vi "Series_ejes_flota.vi"(5 "Tabla_flota":string[][](array[string]), 6 "Tags":string[](array[string])) -> (0 "Nº Ejes":i32[](array[numeric]), 1 "Series del convoy":string[](array[string]), 4 "UT":i32[](array[numeric]))   [LabVIEW 2015]
panel:
  out "Array 2":i32[](array[numeric])
  out "Array":i32[](array[numeric])
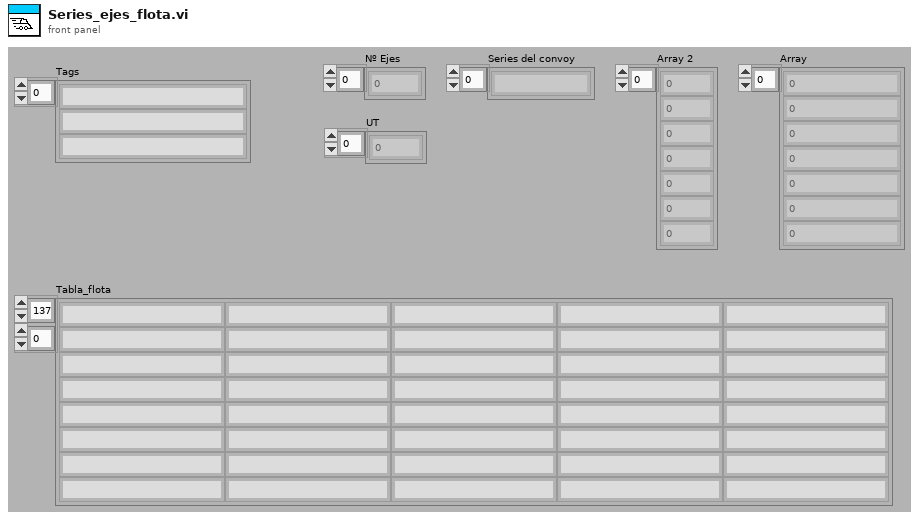
[diagram p1: front panel]
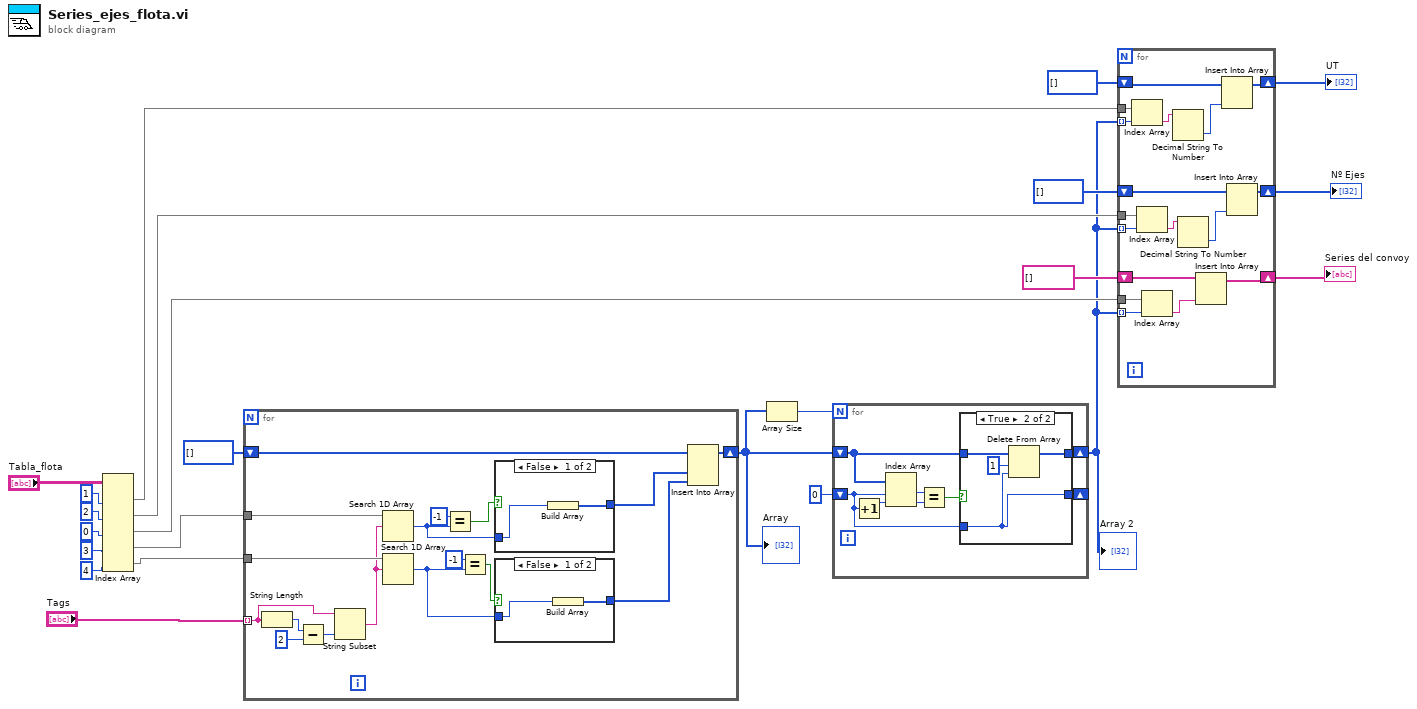
[diagram p0: block diagram]
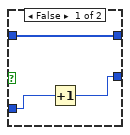
[diagram p2: hidden frame]
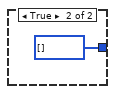
[diagram p3: hidden frame]
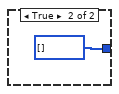
[diagram p4: hidden frame]
diagram:
  n1 = Index Array(array="Tabla_flota", index (col) #1=1 ("index (row)"), index (col) #2=2 ("disabled index (col)"), index (col) #3=0 ("disabled index (col)"), index (col) #4=3 ("disabled index (col)"), index (col) #5=4 ("index (col)")) -> (element #1=w5:string[], element #2=w20:string[], element #3=w17:string[], element #4=w10:string[], element #5=w11:string[])  [unwired: 5 in]
  n2 = for {
    tunnel: "Tags" -> [w28] mode=indexing
    tunnel: w10 -> [w40]
    tunnel: w11 -> [w39]
    shift-right: [w37] -> w13
    shift-left: i32[] [] -> [w38]
    n3 = String Length(string=w28) -> (length=w25:i32)
    n4 = Subtract(x=w25, y=2) -> (x-y=w26:i32)
    n5 = String Subset(string=w28, length (rest)=w26) -> (substring=w27:string)  [unwired: 1 in]
    n6 = Search 1D Array(1D array=w40, element=w27) -> (index of element=w30:i32)  [unwired: 1 in]
    n7 = Search 1D Array(1D array=w39, element=w27) -> (index of element=w29:i32)  [unwired: 1 in]
    n8 = Equal?(x=-1, y=w30) -> (x = y?=w34:bool)
    n9 = Equal?(x=-1, y=w29) -> (x = y?=w33:bool)
    n10 = case shown="False" w34 {
      tunnel: [w44 i32[] []] -> w32
      tunnel: w30 -> [w45 _]
      frame False {
        n11 = Build Array(w45) -> (w44:i32[])
      }
      frame True {
      }
    }
    n12 = case shown="False" w33 {
      tunnel: [w41 i32[] []] -> w31
      tunnel: w29 -> [w42 _]
      frame False {
        n13 = Build Array(w42) -> (w41:i32[])
      }
      frame True {
      }
    }
    n14 = Insert Into Array(array=w38, new element #1=w32, new element #2=w31) -> (w37:i32[])  [unwired: 1 in]
  }
  "Array" <- w13
  n15 = Array Size(array=w13) -> (size(s)=w15:i32)
  n16 = for {
    N: w15 -> [_]
    shift-right: [w50] -> w4
    shift-left: w13 -> [w51]
    shift-right: [w47] -> _
    shift-left: 0 -> [w48]
    n17 = Increment(x=w48) -> (x+1=w49:i32)
    n18 = Index Array(array=w51, index #1=w48, index #2=w49) -> (element #1=w53:i32, element #2=w54:i32)
    n19 = Equal?(x=w53, y=w54) -> (x = y?=w52:bool)
    n20 = case shown="True" w52 {
      tunnel: w51 -> [w57 w61]
      tunnel: [w57 w60] -> w50
      tunnel: w48 -> [w56 w58]
      tunnel: [w55 w58] -> w47
      frame False {
        n21 = Increment(x=w56) -> (x+1=w55:i32)
      }
      frame True {
        n22 = Delete From Array(array=w61, length=1, index=w58) -> (array with subset deleted=w60:i32[])  [unwired: 1 out]
      }
    }
  }
  "Array 2" <- w4
  n23 = for {
    tunnel: w4 -> [w78] mode=indexing
    tunnel: w17 -> [w77]
    shift-right: [w74] -> w23
    shift-left: string[] [] -> [w75]
    tunnel: w20 -> [w73]
    tunnel: w4 -> [w72] mode=indexing
    shift-right: [w70] -> w22
    shift-left: i32[] [] -> [w71]
    shift-right: [w64] -> w3
    shift-left: i32[] [] -> [w65]
    tunnel: w5 -> [w63]
    tunnel: w4 -> [w62] mode=indexing
    n24 = Index Array(array=w63, index=w62) -> (element=w67:string)
    n25 = Index Array(array=w73, index=w72) -> (element=w69:string)
    n26 = Index Array(array=w77, index=w78) -> (element=w76:string)
    n27 = Decimal String To Number(string=w67) -> (number=w66:i32)  [unwired: 2 in, 1 out]
    n28 = Decimal String To Number(string=w69) -> (number=w68:i32)  [unwired: 2 in, 1 out]
    n29 = Insert Into Array(array=w75, new element=w76) -> (w74:string[])  [unwired: 1 in]
    n30 = Insert Into Array(array=w65, new element=w66) -> (w64:i32[])  [unwired: 1 in]
    n31 = Insert Into Array(array=w71, new element=w68) -> (w70:i32[])  [unwired: 1 in]
  }
  "Series del convoy" <- w23
  "Nº Ejes" <- w22
  "UT" <- w3
